vi "PSDATA_Variant To ArrayBool.vi"(9 "error in":errorcluster, 10 "Value":variant) -> (1 "error out":errorcluster, 2 "Value":string, 4 "ArrayBool":bool[](array[boolean]))   [LabVIEW 2016]
doc: "Developer：YDX"
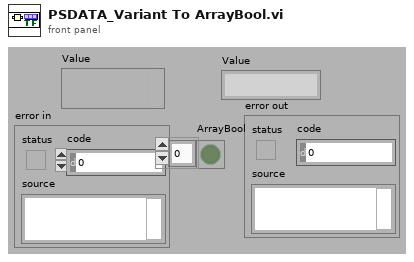
[diagram p1: front panel]
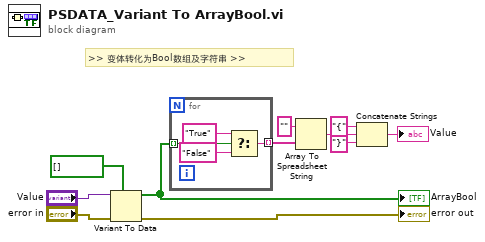
[diagram p0: block diagram]
diagram:
  # ">> 变体转化为Bool数组及字符串 >>"
  n1 = Variant To Data(error in="error in", type=bool[] [], Variant="Value") -> (data=w7:bool[], error out=→"error out":errorcluster)
  "ArrayBool" <- w7
  n2 = for {
    tunnel: [w14] -> w6 mode=indexing
    tunnel: w7 -> [w12] mode=indexing
    n3 = Select(t="True" ("y"), s=w12, f="False") -> (s? t:f=w14:string)
  }
  n4 = Array To Spreadsheet String(array=w6, 3:"" ("format string")) -> (spreadsheet string=w5:string)  [unwired: 1 in]
  n5 = Concatenate Strings("{" ("string"), w5, "}" ("string")) -> (→"Value":string)
